vi "Main Tclk.vi"() -> ()   [LabVIEW 2018] (continued)
            n4773 = event-data() -> ("NewVal"=w4047:bool)  [unwired: 6 out]
            n4774 = case shown="True" w4047 {
              frame False {
              }
              frame True {
                n4775 = stacked-sequence {
                  frame #0 {
                    n4776 = local read "Last milling snapshot"() -> (w4051:path)
                    n4777 = local read "Last FIB recipe"() -> (w4057:path)
                    n4778 = local read "Re-engage Files"() -> (w4063:path)
                    n4779 = File/Directory Info(path=w4057) -> (path out=w4056:path, error out=w4052:errorcluster)  [unwired: 1 in, 5 out]
                    n4780 = Build Path(base path=w4063, name or relative path="pre.png") -> (appended path=w4061:path)
                    n4781 = File/Directory Info(path=w4051) -> (path out=w4050:path, error out=w4048:errorcluster)  [unwired: 1 in, 5 out]
                    n4782 = Unbundle By Name(w4052) -> ("status"=w4053:bool)
                    n4783 = Unbundle By Name(w4048) -> ("status"=w4049:bool)
                    n4784 = File/Directory Info(path=w4061) -> (error out=w4058:errorcluster)  [unwired: 1 in, 6 out]
                    n4785 = case shown="False" w4049 {
                      tunnel: w4050 -> [w4066 _]
                      tunnel: [w4065 w4069] -> w4060
                      tunnel: w4048 -> [_ w4069]
                      frame False {
                        n4786 = call-poly <vilib>:"Read From XML File.vi"("XML File Path"=w4066) -> ("error out"=w4064:errorcluster, "XML Elements"=w4067:string)  [unwired: 8 in, 1 out]
                        n4787 = Unflatten From XML(xml string=w4067, type=T47 {"Timestamp"=timestamp(0 s since 1904-01-01), "Double"=0.0, "FIB slice #"=0, "Reheat"=FALSE, "Double 2"=0.0, "Double 3"=0.0, "Double 4"=0.0} ("output cluster"), error in (no error)=w4064) -> (error out=w4065:errorcluster)  [unwired: 1 out]
                      }
                      frame True {
                      }
                    }
                    n4788 = case shown="False" w4053 {
                      tunnel: [w4071 w4073] -> w4059
                      tunnel: w4056 -> [w4070 _]
                      tunnel: w4052 -> [_ w4073]
                      frame False {
                        n4789 = call "Recipe read write.vi"("Write"=FALSE, "Recipe path"=w4070) -> ("error out"=w4071:errorcluster)  [unwired: 6 in, 3 out]
                      }
                      frame True {
                      }
                    }
                    n4790 = Merge Errors(w4060, w4059, w4058) -> (w4054:errorcluster)
                    n4791 = Unbundle By Name(w4054) -> ("status"=w4055:bool)
                    n4792 = local write "error out"(w4054) -> ()
                    n4793 = case shown="True" w4055 {
                      frame False {
                      }
                      frame True {
                        n4794 = local read "Milling para"() -> (w4076:T35)
                        n4795 = Two Button Dialog(message="Files needed for resume do not exist or are corrupted\nLoad information from the last good data file (*.dat)?") -> (T button?=w4074:bool)  [unwired: 2 in]
                        "dat to csv and xml" <- w4074
                        n4796 = Bundle By Name(cluster=w4076, "Mill start from Last"=w4074) -> (w4075:T35)
                        n4797 = local write "Milling para"(w4075) -> ()
                      }
                    }
                  }
                  frame #1 {
                    n4798 = local read "dat to csv and xml"() -> (w4078:bool)
                    n4799 = case shown="True" w4078 {
                      frame False {
                      }
                      frame True {
                        n4800 = call "File Dialog4"("start path"=path "E:/Images", "prompt"="Select the last good .dat file", "pattern (all files)"="*.dat" ("pattern label"), "pattern label"="Data file") -> ("selected path"=w4081:path, "cancelled"=w4079:bool, "error out"=w4084:errorcluster)  [unwired: 8 in, 1 out]
                        n4801 = local write "Read recipe path"(w4081) -> ()
                        n4802 = local write "error out"(w4084) -> ()
                        n4803 = case shown="True" w4079 {
                          frame False {
                            n4804 = local write "Load recipe"(TRUE ("Load recipe")) -> ()
                          }
                          frame True {
                            n4805 = local read "Milling para"() -> (w4087:T35)
                            n4806 = Bundle By Name(cluster=w4087, "Mill start from Last"=FALSE) -> (w4089:T35)
                            n4807 = local write "Milling para"(w4089) -> ()
                          }
                        }
                      }
                    }
                  }
                  frame #2 {
                    n4808 = local read "Milling para"() -> (w4091:T35)
                    n4809 = Unbundle By Name(w4091) -> ("Mill start from Last"=w4090:bool)
                    n4810 = case shown="True" w4090 {
                      frame False {
                      }
                      frame True {
                        n4811 = One Button Dialog(message="Resume from the last recipe and milling position ") -> ()  [unwired: 1 in, 1 out]
                      }
                    }
                  }
                }
              }
            }
          }
          event "Milling para.FIB PID reset": Value Change {
            n4812 = event-data() -> ("NewVal"=w4093:bool)  [unwired: 2 out]
            n4813 = shared-variable ".\\Zeiss Library.lvlib\\FIB PID reset"(w4093) -> ()  [unwired: 1 in, 1 out]
          }
          event "Milling para.FIB PID target": Value Change {
            n4814 = event-data() -> ()  [unwired: 7 out]
            n4815 = local read "Alert Settings"() -> (w4096:T36)
            n4816 = Bundle By Name(cluster=w4096, "FIB CL current alarm"=FALSE) -> (w4095:T36)
            n4817 = local write "Alert Settings"(w4095) -> ()
          }
          event "Pre image": Value Change {
            n4818 = event-data() -> ("NewVal"=w4097:bool)  [unwired: 2 out]
            n4819 = case shown="True" w4097 {
              frame False {
                n4820 = local write "Status message"("standby" ("Status message")) -> ()
                n4821 = shared-variable "My Computer\\Zeiss Library.lvlib\\Realtime Imaging stop"(TRUE ("Unfreeze")) -> ()  [unwired: 1 in, 1 out]
              }
              frame True {
                n4822 = stacked-sequence {
                  frame #0 {
                    n4823 = local read "FIB HW Config"() -> (w4108:T23)
                    n4824 = local read "FIB HW Config"() -> (w4105:T23)
                    n4825 = local write "Status message"("FIB Pre Imaging" ("Status message")) -> ()
                    n4826 = Unbundle By Name(w4108) -> ("Beam blank"=w4107:tag)
                    n4827 = Unbundle By Name(w4105) -> ("FIB Ext Scan"=w4103:tag)
                    n4828 = local read "Api"() -> (w4100:refnum<k7>)
                    n4829 = call "FIB beam blank.vi"("Api"=w4100, "Beam blanked"=TRUE, "lines"=w4107) -> ()  [unwired: 2 in, 1 out]
                    n4830 = call "FIB ext scan.vi"("Ext on"=TRUE ("data"), "FIB Ext Scan"=w4103) -> ()  [unwired: 9 in, 1 out]
                    n4831 = local write "Image Tabs"(T37."FIB Milling Offset after Pause" ("Image Tabs")) -> ()
                  }
                  frame #1 {
                    n4832 = local read "Machine Type"() -> (w4109:u8)
                    n4833 = case shown="1" w4109 {
                      frame 0, Default {
                      }
                      frame 1 {
                        w4112 = TRUE ("Close session")
                        n4834 = local read "COM port"() -> (w4114:refnum<visa-resource-name>)
                        n4835 = call "Remcon32 command.vi"("Initialization"=w4112, "SEM command"="edx 1", "COM port in"=w4114) -> ("COM port out"=w4113:refnum<visa-resource-name>)  [unwired: 5 in, 3 out]
                        n4836 = call "FIB mode.vi"("Close session"=w4112, "Iterations"=u32 3, "FIB mode"=T10."FIB", "COM port in"=w4113) -> ()  [unwired: 6 in, 2 out]
                      }
                    }
                  }
                  frame #2 {
                    n4837 = shared-variable ".\\Zeiss Library.lvlib\\Milling Z Voltage RT"() -> (w4117:sgl)  [unwired: 1 in, 1 out]
                    n4838 = local read "FIB Options"() -> (w4120:T33)
                    n4839 = local read "FIB Scan Parameters"() -> (w4124:T32)
                    n4840 = property on="Pre Image" class="IntGraph (strict)"() -> ("Width"=w4133:u32, "Height"=w4132:u32)  [unwired: 2 in, 2 out]
                    n4841 = local read "FIB Options"() -> (w4140:T33)
                    n4842 = local read "Milling para"() -> (w4123:T35)
                    n4843 = local read "FIB Scan Parameters"() -> (w4146:T32)
                    n4844 = expression code="x/1000"("FIB Y zoom pixel (nm)") -> (w4134:dbl)
                    n4845 = Decrement(x=w4132) -> (x-1=w4131:u32)
                    n4846 = Unbundle By Name(w4120) -> ("Flip z"=w4119:bool)
                    n4847 = Unbundle By Name(w4140) -> ("Flip x"=w4136:bool)
                    n4848 = Unbundle By Name(w4123) -> ("X offset (um)"=w4152:sgl, "X center (um)"=w4151:sgl, "FIB FOV (um)"=w4122:sgl)
                    n4849 = Multiply(x=w4134, y=w4131) -> (x*y=w4130:dbl)
                    "FIB Y zoom size (um)" <- w4130
                    n4850 = Unbundle By Name(w4124) -> ("Z size (V)"=w4125:dbl)
                    n4851 = Unbundle By Name(w4146) -> ("X size (V)"=w4141:dbl)
                    n4852 = Negate(x=w4117) -> (-x=w4118:sgl)
                    n4853 = Add(x=w4152, y=w4151) -> (x+y=w4153:sgl)
                    n4854 = Select(t=w4118, s=w4119, f=w4117) -> (s? t:f=w4116:sgl)
                    n4855 = Divide(x=w4116, y=w4125) -> (x/y=w4126:dbl)
                    n4856 = Multiply(x=w4126, y=w4122) -> (x*y=w4127:dbl)
                    n4857 = shared-variable ".\\Zeiss Library.lvlib\\Milling Z Voltage RT"() -> (w4149:sgl)  [unwired: 1 in, 1 out]
                    n4858 = call "Milling parameter to trapezoidal shape.vi"("Y location (um)"=w4127, "Milling para"=w4123) -> ("X size (um) @ Y"=w4121:dbl)  [unwired: 5 in, 4 out]
                    n4859 = expression code="x*1.2"(w4121) -> (w4128:dbl)
                    "FIB X zoom size (um)" <- w4128
                    n4860 = Divide(x=w4153, y=w4122) -> (x/y=w4142:sgl)
                    n4861 = Divide(x=w4128, y=w4122) -> (x/y=w4145:dbl)
                    n4862 = Multiply(x=w4142, y=w4141) -> (x*y=w4138:dbl)
                    n4863 = Multiply(x=w4145, y=w4141) -> (x*y=w4129:dbl)
                    n4864 = Multiply(x=w4141, y=w4130) -> (x*y=w4144:dbl)
                    n4865 = Negate(x=w4138) -> (-x=w4139:dbl)
                    n4866 = Divide(x=w4144, y=w4122) -> (x/y=w4143:dbl)
                    n4867 = Select(t=w4139, s=w4136, f=w4138) -> (s? t:f=w4137:dbl)
                    n4868 = local read "FIB Zoom Parameters"() -> (w4155:T34)
                    n4869 = Bundle By Name(cluster=w4155, "X resolution"=w4133, "Y resolution"=w4131, "X center"=w4137, "X size (V)"=w4129, "Y center"=w4149, "Y size (V)"=w4143, "Frame line rampdown ratio"=-0.1, "Scan rate (Hz)"=u32 200000, "Oversampling"=u16 20) -> (w4154:T34)
                    n4870 = local write "FIB Zoom Parameters"(w4154) -> ()
                  }
                  frame #3 {
                    n4871 = Wait (ms)(milliseconds to wait=u32 200) -> ()  [unwired: 1 out]
                  }
                  frame #4 {
                    w4158 = TRUE ("As subVi")
                    n4872 = local read "FIB HW Config"() -> (w4159:T23)
                    n4873 = local read "FIB Options"() -> (w4160:T33)
                    n4874 = call "FIB realtime imaging PXIe-6124.vi"("HW Config"=w4159, "Options"=w4160, "Single scan"=w4158, "Scan Para"="FIB Zoom Parameters", "As subVi"=w4158) -> ()  [unwired: 4 in, 2 out]
                  }
                  frame #5 {
                    n4875 = Wait (ms)(milliseconds to wait=u32 100) -> ()  [unwired: 1 out]
                    n4876 = local read "Milling para"() -> (w4166:T35)
                    n4877 = local read "FIB Zoom Parameters"() -> (w4161:T34)
                    n4878 = control-ref of="Pre Image"() -> (w4169:refnum<vi>)
                    n4879 = local read "FIB Scan Parameters"() -> (w4164:T32)
                    n4880 = local read "FIB Options"() -> (w4163:T33)
                    n4881 = shared-variable ".\\Zeiss Library.lvlib\\Milling Z Voltage RT"() -> (w4162:sgl)  [unwired: 1 in, 1 out]
                    n4882 = call "FIB zoom image draw milling.vi"("Milling Z voltage"=w4162, "Milling para"=w4166, "FIB Zoom Parameters"=w4161, "FIB Options"=w4163, "FIB Scan Parameters"=w4164, "Pre image"=TRUE, "Image reference"=w4169) -> ()  [unwired: 5 in]
                    n4883 = Unbundle By Name(w4166) -> ("X offset (um)"=→"X offset pre (um)":sgl, "Z offset (um)"=→"Y offset pre (um)":sgl)
                  }
                  frame #6 {
                    n4884 = local read "Pre Image"() -> (w4171:i16[][])
                    n4885 = Array Size(array=w4171) -> (size(s)=w4172:i32[])
                    n4886 = local write "Pre image"(FALSE ("Pre image")) -> ()
                    n4887 = local write "Status message"("standby" ("Status message")) -> ()
                    n4888 = Add Array Elements(numeric array=w4172) -> (sum=w4173:i32)
                    n4889 = Not Equal To 0?(x=w4173) -> (x != 0?=w4174:bool)
                    n4890 = case shown="True" w4174 {
                      tunnel: w4171 -> [_ w4179]
                      frame False {
                      }
                      frame True {
                        n4891 = local read "Last FIB zoom pre image"() -> (w4181:path)
                        n4892 = call "16bit Image Normalization.vi"("Transpose"=FALSE, "Input image"=w4179) -> ("Normalized image"=w4178:u8[][])  [unwired: 5 in, 4 out]
                        n4893 = call <vilib>:"Flatten Pixmap.vi"("colors"=u32[] [16777222, 65793, 131586, 197379, 263172, 328965, 394758, 460551, 526344, 592137, 657930, 723723, 789516, 855309, 921102, 986895, 1052688, 1118481, 1184274, 1250067, 1315860, 1381653, 1447446, 1513239, 1579032, 1644825, 1710618, 1776411, 1842204, 1907997, 1973790, 2039583, 2105376, 2171169, 2236962, 2302755, 2368548, 2434341, 2500134, 2565927, 2631720, 2697513, 2763306, 2829099, 2894892, 2960685, 3026478, 3092271, 3158064, 3223857, 3289650, 3355443, 3421236, 3487029, 3552822, 3618615, 3684408, 3750201, 3815994, 3881787, 3947580, 4013373, 4079166, 4144959, 4210752, 4276545, 4342338, 4408131, 4473924, 4539717, 4605510, 4671303, 4737096, 4802889, 4868682, 4934475, 5000268, 5066061, 5131854, 5197647, 5263440, 5329233, 5395026, 5460819, 5526612, 5592405, 5658198, 5723991, 5789784, 5855577, 5921370, 5987163, 6052956, 6118749, 6184542, 6250335, 6316128, 6381921, 6447714, 6513507, 6579300, 6645093, 6710886, 6776679, 6842472, 6908265, 6974058, 7039851, 7105644, 7171437, 7237230, 7303023, 7368816, 7434609, 7500402, 7566195, 7631988, 7697781, 7763574, 7829367, 7895160, 7960953, 8026746, 8092539, 8158332, 8224125, 8289918, 8355711, 8421504, 8487297, 8553090, 8618883, 8684676, 8750469, 8816262, 8882055, 8947848, 9013641, 9079434, 9145227, 9211020, 9276813, 9342606, 9408399, 9474192, 9539985, 9605778, 9671571, 9737364, 9803157, 9868950, 9934743, 10000536, 10066329, 10132122, 10197915, 10263708, 10329501, 10395294, 10461087, 10526880, 10592673, 10658466, 10724259, 10790052, 10855845, 10921638, 10987431, 11053224, 11119017, 11184810, 11250603, 11316396, 11382189, 11447982, 11513775, 11579568, 11645361, 11711154, 11776947, 11842740, 11908533, 11974326, 12040119, 12105912, 12171705, 12237498, 12303291, 12369084, 12434877, 12500670, 12566463, 12632256, 12698049, 12763842, 12829635, 12895428, 12961221, 13027014, 13092807, 13158600, 13224393, 13290186, 13355979, 13421772, 13487565, 13553358, 13619151, 13684944, 13750737, 13816530, 13882323, 13948116, 14013909, 14079702, 14145495, 14211288, 14277081, 14342874, 14408667, 14474460, 14540253, 14606046, 14671839, 14737632, 14803425, 14869218, 14935011, 15000804, 15066597, 15132390, 15198183, 15263976, 15329769, 15395562, 15461355, 15527148, 15592941, 15658734, 15724527, 15790320, 15856113, 15921906, 15987699, 16053492, 16119285, 16185078, 16250871, 16316664, 16382457, 16448250, 16514043, 16579836, 16645629, 16711422, 16448250] ("256 gray scale"), "8-bit pixmap"=w4178) -> ("image data"=w4180:T55)  [unwired: 4 in, 5 out]
                        n4894 = call <vilib>:"Write PNG File.vi"("image data"=w4180, "path to PNG file"=w4181) -> ()  [unwired: 1 in, 9 out]
                      }
                    }
                  }
                }
              }
            }
          }
          event "Post image": Value Change {
            n4895 = event-data() -> ("NewVal"=w4183:bool)  [unwired: 2 out]
            n4896 = case shown="True" w4183 {
              frame False {
                n4897 = local write "Status message"("standby" ("Status message")) -> ()
                n4898 = shared-variable "My Computer\\Zeiss Library.lvlib\\Realtime Imaging stop"(TRUE ("Unfreeze")) -> ()  [unwired: 1 in, 1 out]
              }
              frame True {
                n4899 = stacked-sequence {
                  frame #0 {
                    n4900 = local read "FIB HW Config"() -> (w4194:T23)
                    n4901 = local read "FIB HW Config"() -> (w4191:T23)
                    n4902 = local write "Status message"("FIB Post Imaging" ("Status message")) -> ()
                    n4903 = Unbundle By Name(w4194) -> ("Beam blank"=w4193:tag)
                    n4904 = Unbundle By Name(w4191) -> ("FIB Ext Scan"=w4189:tag)
                    n4905 = local read "Api"() -> (w4186:refnum<k7>)
                    n4906 = call "FIB beam blank.vi"("Api"=w4186, "Beam blanked"=TRUE, "lines"=w4193) -> ()  [unwired: 2 in, 1 out]
                    n4907 = call "FIB ext scan.vi"("Ext on"=TRUE ("data"), "FIB Ext Scan"=w4189) -> ()  [unwired: 9 in, 1 out]
                    n4908 = local write "Image Tabs"(T37."FIB Milling Offset after Pause" ("Image Tabs")) -> ()
                  }
                  frame #1 {
                    n4909 = local read "Machine Type"() -> (w4195:u8)
                    n4910 = case shown="1" w4195 {
                      frame 0, Default {
                      }
                      frame 1 {
                        w4198 = TRUE ("Close session")
                        n4911 = local read "COM port"() -> (w4200:refnum<visa-resource-name>)
                        n4912 = call "Remcon32 command.vi"("Initialization"=w4198, "SEM command"="edx 1", "COM port in"=w4200) -> ("COM port out"=w4199:refnum<visa-resource-name>)  [unwired: 5 in, 3 out]
                        n4913 = call "FIB mode.vi"("Close session"=w4198, "Iterations"=u32 3, "FIB mode"=T10."FIB", "COM port in"=w4199) -> ()  [unwired: 6 in, 2 out]
                      }
                    }
                  }
                  frame #2 {
                    n4914 = local read "FIB Y zoom pixel (nm)"() -> (w4222:dbl)
                    n4915 = property on="Pre Image" class="IntGraph (strict)"() -> ("Height"=w4221:u32)  [unwired: 2 in, 2 out]
                    n4916 = local read "FIB Scan Parameters"() -> (w4218:T32)
                    n4917 = local read "Milling para"() -> (w4219:T35)
                    n4918 = local read "FIB Zoom Parameters"() -> (w4204:T34)
                    n4919 = shared-variable ".\\Zeiss Library.lvlib\\Milling Z Voltage RT"() -> (w4203:sgl)  [unwired: 1 in, 1 out]
                    n4920 = Decrement(x=w4221) -> (x-1=w4212:u32)
                    n4921 = Unbundle By Name(w4219) -> ("FIB FOV (um)"=w4220:sgl)
                    n4922 = Unbundle By Name(w4218) -> ("X size (V)"=w4217:dbl)
                    n4923 = expression code="x/1000"(w4222) -> (w4213:dbl)
                    n4924 = Unbundle By Name(w4204) -> ("Y size (V)"=w4209:dbl)
                    n4925 = Bundle By Name(cluster=w4204, "Y center"=w4203) -> (w4202:T34)
                    n4926 = Multiply(x=w4212, y=w4217) -> (x*y=w4216:dbl)
                    n4927 = Divide(x=w4216, y=w4220) -> (x/y=w4215:dbl)
                    n4928 = local write "FIB Zoom Parameters"(w4202) -> ()
                    n4929 = Divide(x=w4209, y=w4215) -> (x/y=w4214:dbl)
                    n4930 = Multiply(x=w4213, y=w4215) -> (x*y=w4210:dbl)
                    n4931 = Subtract(x=w4210, y=w4209) -> (x-y=w4206:dbl)
                    n4932 = Multiply(x=w4213, y=w4212) -> (x*y=w4211:dbl)
                    n4933 = Absolute Value(x=w4206) -> (abs(x)=w4205:dbl)
                    n4934 = Greater?(x=w4205, y=0.0001) -> (0:w4208:bool)
                    n4935 = case shown="True" w4208 {
                      tunnel: w4210 -> [_ w4228]
                      tunnel: w4214 -> [_ w4225]
                      tunnel: w4211 -> [_ w4223]
                      frame False {
                      }
                      frame True {
                        n4936 = expression code="x*1000"(w4225) -> (w4224:dbl)
                        n4937 = Two Button Dialog(message="Y pixel was modified since the last pre image was taken", 1:"Continue with new value" ("T button name (\"OK\")"), 2:"Use old value" ("T button name (\"OK\")")) -> (T button?=w4229:bool)
                        n4938 = case shown="True" w4229 {
                          tunnel: w4228 -> [w4232 _]
                          tunnel: w4224 -> [_ w4235]
                          tunnel: w4223 -> [w4231 _]
                          frame False {
                            n4939 = local read "FIB Zoom Parameters"() -> (w4234:T34)
                            n4940 = Bundle By Name(cluster=w4234, "Y size (V)"=w4232) -> (w4233:T34)
                            n4941 = local write "FIB Zoom Parameters"(w4233) -> ()
                            n4942 = local write "FIB Y zoom size (um)"(w4231) -> ()
                          }
                          frame True {
                            n4943 = local write "FIB Y zoom pixel (nm)"(w4235) -> ()
                          }
                        }
                      }
                    }
                  }
                  frame #3 {
                    w4237 = TRUE ("As subVi")
                    n4944 = local read "FIB Zoom Parameters"() -> (w4236:T34)
                    n4945 = local read "FIB HW Config"() -> (w4238:T23)
                    n4946 = local read "FIB Options"() -> (w4239:T33)
                    n4947 = call "FIB realtime imaging PXIe-6124.vi"("HW Config"=w4238, "Options"=w4239, "Single scan"=w4237, "Scan Para"=w4236, "As subVi"=w4237) -> ()  [unwired: 4 in, 2 out]
                  }
                  frame #4 {
                    n4948 = Wait (ms)(milliseconds to wait=u32 100) -> ()  [unwired: 1 out]
                  }
                  frame #5 {
                    n4949 = local read "FIB Zoom Parameters"() -> (w4266:T34)
                    n4950 = local read "X offset pre (um)"() -> (w4242:dbl)
                    n4951 = local read "Y offset pre (um)"() -> (w4241:dbl)
                    n4952 = local read "Post Image"() -> (w4255:i16[][])
                    n4953 = local read "Pre Image"() -> (w4254:i16[][])
                    n4954 = call "Image Alignment.vi"("Image 2"=w4254, "Image 1"=w4255) -> ("Y shift"=w4258:i32, "X shift"=w4263:i32)  [unwired: 7 in, 1 out]
                    n4955 = Unbundle By Name(w4266) -> ("X resolution"=w4262:u32, "Y resolution"=w4257:u32, "X size (V)"=w4261:dbl, "Y size (V)"=w4256:dbl)
                    n4956 = Divide(x=w4263, y=w4262) -> (x/y=w4259:dbl)
                    n4957 = Divide(x=w4258, y=w4257) -> (x/y=w4260:dbl)
                    n4958 = local read "Milling para"() -> (w4265:T35)
                    n4959 = local read "FIB Scan Parameters"() -> (w4264:T32)
                    n4960 = Multiply(x=w4259, y=w4261) -> (x*y=w4250:dbl)
                    n4961 = Multiply(x=w4260, y=w4256) -> (x*y=w4251:dbl)
                    n4962 = Unbundle By Name(w4265) -> ("FIB FOV (um)"=w4253:sgl)
                    n4963 = Unbundle By Name(w4264) -> ("X size (V)"=w4252:dbl)
                    n4964 = Divide(x=w4253, y=w4252) -> (x/y=w4249:dbl)
                    n4965 = Multiply(x=w4250, y=w4249) -> (x*y=w4246:dbl)
                    n4966 = Multiply(x=w4251, y=w4249) -> (x*y=w4244:dbl)
                    n4967 = Add(x=w4246, y=w4242) -> (x+y=w4245:dbl)
                    n4968 = Add(x=w4244, y=w4241) -> (x+y=w4243:dbl)
                    n4969 = local read "Milling para"() -> (w4248:T35)
                    n4970 = Bundle By Name(cluster=w4248, "X offset (um)"=w4245, "Z offset (um)"=w4243) -> (w4247:T35)
                    n4971 = local write "Milling para"(w4247) -> ()
                  }
                  frame #6 {
                    n4972 = local read "X offset pre (um)"() -> (w4269:dbl)
                    n4973 = local read "Y offset pre (um)"() -> (w4268:dbl)
                    n4974 = local read "Milling para"() -> (w4274:T35)
                    n4975 = local read "FIB Zoom Parameters"() -> (w4267:T34)
                    n4976 = control-ref of="Post Image"() -> (w4275:refnum<vi>)
                    n4977 = local read "FIB Scan Parameters"() -> (w4272:T32)
                    n4978 = local read "FIB Options"() -> (w4271:T33)
                    n4979 = shared-variable ".\\Zeiss Library.lvlib\\Milling Z Voltage RT"() -> (w4270:sgl)  [unwired: 1 in, 1 out]
                    n4980 = call "FIB zoom image draw milling.vi"("Milling Z voltage"=w4270, "Milling para"=w4274, "Z offset pre (um)"=w4268, "X offset pre (um)"=w4269, "FIB Zoom Parameters"=w4267, "FIB Options"=w4271, "FIB Scan Parameters"=w4272, "Pre image"=FALSE, "Image reference"=w4275) -> ()  [unwired: 3 in]
                  }
                  frame #7 {
                    n4981 = local write "Post image"(FALSE ("Pre image")) -> ()
                    n4982 = local write "Status message"("standby" ("Status message")) -> ()
                  }
                }
              }
            }
          }
          event "Hardware Configuration.Save config file": Value Change {
            # "THIS VI WRITES ALL THE HARDWARE CONFIG TAB CONTROLS TO THE .INI FILE."
            n4983 = event-data() -> ()  [unwired: 2 out]
            n4984 = disable-structure shown="Disabled" {
              frame Disabled {
                n4985 = stacked-sequence {
                  frame #0 {
                    n4986 = local read "HW config items"() -> (w4281:string[])
                    n4987 = local read "Hardware Configuration"() -> (w4285:T25)
                    n4988 = local read "Detector Information"() -> (w4286:T8)
                    n4989 = local read "Hardware Configuration"() -> (w4283:T25)
                    n4990 = Unbundle By Name(w4285) -> ("Machine ID"=w4294:string, "Machine Type"=w4300:u8, "SEM Max FOV (um)"=w4287:sgl, "Det min (V)"=w4288:dbl, "Det max (V)"=w4289:dbl)
                    n4991 = Unbundle By Name(w4286) -> ("Brightness A"=w4291:dbl, "Contrast A"=w4290:dbl, "Detector B name"=w4295:string, "Brightness B"=w4292:dbl, "Contrast B"=w4293:dbl)
                    n4992 = Unbundle By Name(w4283) -> ("Configuration file"=w4282:path)
                    n4993 = Build Array(w4287, w4288, w4289, w4291, w4290) -> (w4296:dbl[])
                    n4994 = Build Array(w4292, w4293) -> (w4298:dbl[])
                    n4995 = case shown="2" w4300 {
                      tunnel: ["Feiss" ("Machine ID") "NVision" ("Machine ID") "Jeiss" ("Machine ID")] -> w4301
                      frame 0, Default {
                      }
                      frame 1 {
                      }
                      frame 2 {
                      }
                    }
                    n4996 = for {
                      tunnel: w4296 -> [w4322] mode=indexing
                      tunnel: [w4321] -> w4297 mode=indexing
                      n4997 = Format Into String(w4322) -> (resulting string=w4321:string)  [unwired: 3 in, 1 out]
                    }
                    n4998 = for {
                      tunnel: w4298 -> [w4320] mode=indexing
                      tunnel: [w4319] -> w4299 mode=indexing
                      n4999 = Format Into String(w4320) -> (resulting string=w4319:string)  [unwired: 3 in, 1 out]
                    }
                    n5000 = Build Array (concatenate)(w4294, w4301, w4297, w4295, w4299) -> (w4302:string[])
                    n5001 = for {
                      tunnel: w4281 -> [w4315] mode=indexing
                      tunnel: w4302 -> [w4313] mode=indexing
                      tunnel: [w4312] -> w4284 mode=indexing
                      n5002 = Concatenate Strings(w4315, "," ("string"), w4313) -> (w4312:string)
                    }
                    n5003 = Build Path(name or relative path=w4282) -> (appended path=w4305:path)  [unwired: 1 in]
                    n5004 = Open/Create/Replace File(file path (use dialog)=w4305, operation (0:open)=T49."replace or create with confirmation") -> (refnum out=w4307:refnum<file>, error out=w4308:errorcluster)  [unwired: 1 in, 4 out]
                    n5005 = Set File Position(refnum=w4307, from (0:start)=enum16{"start", "end", "current"}."end", error in=w4308) -> (refnum out=w4309:refnum<file>, error out=w4306:errorcluster)  [unwired: 1 out]
                    n5006 = Write to Text File(file (use dialog)=w4309, text=w4284, error in=w4306) -> (refnum out=w4310:refnum<file>, error out=w4311:errorcluster)  [unwired: 2 out]
                    n5007 = Close File(refnum=w4310, error in=w4311) -> ()  [unwired: 2 out]
                  }
                  frame #1 {
                    n5008 = local read "Hardware Configuration"() -> (w4325:T25)
                    n5009 = Bundle By Name(cluster=w4325, "Save config file"=FALSE) -> (w4324:T25)
                    n5010 = local write "Hardware Configuration"(w4324) -> ()
                  }
                }
              }
              frame Enabled {
              }
            }
            n5011 = local read "Hardware Configuration"() -> (w4280:T25)
            n5012 = Bundle By Name(cluster=w4280, "Save config file"=FALSE) -> (w4279:T25)
            n5013 = local write "Hardware Configuration"(w4279) -> ()
            n5014 = call "Write Config Settings to INI file.vi"("Hardware Configuration"=w4279) -> ()  [unwired: 11 in]
          }
          event "File Information.Save recipe": Value Change {
            n5015 = event-data() -> ()  [unwired: 2 out]
            n5016 = stacked-sequence {
              frame #0 {
              }
              frame #1 {
                n5017 = call "File Dialog"("start path"=path "E:/Recipes", "prompt"="Select an existing recipe to \noverwrite or a directory for \nthe new recipe") -> ("selected path"=w4328:path, "cancelled"=w4330:bool, "error out"=→"error out":errorcluster)  [unwired: 10 in, 1 out]
                n5018 = case shown="False" w4330 {
                  tunnel: w4328 -> [w4337 _]
                  frame False {
                    n5019 = Strip Path(path=w4337) -> (name=w4333:string)  [unwired: 1 out]
                    n5020 = xnode "Match Regular Expression"("input string"=w4333, "regular expression"=".csv") -> ("offset past match"=w4335:i32)  [unwired: 4 in, 4 out]
                    n5021 = Equal?(x=w4335, y=-1) -> (x = y?=w4334:bool)
                    n5022 = case shown="True" w4334 {
                      tunnel: [w4340 w4341] -> w4339
                      tunnel: w4333 -> [w4340 _]
                      frame False {
                      }
                      frame True {
                        n5023 = call "Recipe File Name"() -> ("FIB-SEM recipe YY-MM-DD <user input>.csv"=w4341:string)  [unwired: 17 in, 2 out]
                      }
                    }
                    n5024 = local read "Recipe input"() -> (w4331:T7)
                    n5025 = call "Recipe read write.vi"("Write"=TRUE, "Info"=w4339, "Recipe path"=w4337, "Write input"=w4331) -> ()  [unwired: 4 in, 4 out]
                  }
                  frame True {
                  }
                }
              }
              frame #2 {
                n5026 = Wait (ms)(milliseconds to wait=u32 200) -> ()  [unwired: 1 out]
              }
              frame #3 {
                n5027 = local read "File Information"() -> (w4456:T31)
                n5028 = Bundle By Name(cluster=w4456, "Save recipe"=FALSE ("Save config file")) -> (w4455:T31)
                n5029 = local write "File Information"(w4455) -> ()
              }
            }
          }
          event "File Information.Load recipe": Value Change {
            n5030 = event-data() -> ()  [unwired: 2 out]
            n5031 = stacked-sequence {
              tunnel: [w4460 _ _] -> w4458
              tunnel: w4457 -> [w4459 _ _]
              frame #0 {
                n5032 = call "File Dialog2"("start path"=path "E:/images", "prompt"="Select the recipe", "pattern (all files)"="*.csv;*.dat" ("pattern label"), "pattern label"="Recipe or Data file") -> ("selected path"=w4464:path, "cancelled"=w4465:bool, "error out"=w4466:errorcluster)  [unwired: 8 in, 1 out]
                n5033 = local write "error out"(w4466) -> ()
                n5034 = case shown="False" w4465 {
                  tunnel: w4464 -> [w4469 _]
                  tunnel: [w4468 w4497] -> w4460
                  tunnel: w4459 -> [_ w4497]
                  frame False {
                    n5035 = stacked-sequence {
                      tunnel: w4469 -> [w4471 _ _]
                      tunnel: [_ _ w4496] -> w4468
                      frame #0 {
                        n5036 = local write "Read recipe path"(w4471) -> ()
                        n5037 = Strip Path(path=w4471) -> (name=w4474:string)  [unwired: 1 out]
                        n5038 = Match Pattern(string=w4474, regular expression=".dat") -> (offset past match=w4473:i32)  [unwired: 1 in, 3 out]
                        n5039 = Not Equal?(x=w4473, y=-1) -> (x != y?=w4470:bool)
                        n5040 = case shown="True" w4470 {
                          tunnel: w4471 -> [_ w4493]
                          frame False {
                          }
                          frame True {
                            n5041 = call "Zeiss File Header Tclk.vi"("Write"=FALSE, "Input file path"=w4493) -> ("Ouputs"=w4492:T79)  [unwired: 7 in, 2 out]
                            n5042 = Unbundle By Name(w4492) -> ("SEM parameters"=w4491:T13, "FIB parameters"=w4490:T80, "Data Logging"=w4488:T81)
                            n5043 = Unbundle By Name(w4488) -> ("Temp (F)"=w4487:sgl, "FIB Faraday Cup (nA)"=w4486:sgl, "FIB Specimen I (nA)"=w4485:sgl, "Beam Dump 1 (nA)"=w4484:sgl, "Beam Dump 2 (nA)"=w4477:sgl, "Milling I (nA)"=w4476:sgl, "SEM Specimen I (nA)"=w4479:sgl, "Milling Z voltage (V)"=w4483:sgl, "Focus Index"=w4482:sgl, "FIB slice #"=w4481:u32)
                            n5044 = local write "SEM Parameters"(w4491) -> ()
                            n5045 = local write "FIB Parameters"(w4490) -> ()
                            n5046 = local write "Temp (F)"(w4487) -> ()
                            n5047 = local write "Faraday Cup (nA)"(w4486) -> ()
                            n5048 = local write "Specimen I (nA)"(w4485) -> ()
                            n5049 = local write "Beam Dump 1 (nA)"(w4484) -> ()
                            n5050 = local write "Beam Dump 2 (nA)"(w4477) -> ()
                            n5051 = local write "Milling I (nA)"(w4476) -> ()
                            n5052 = local write "Milling Z voltage (V)"(w4483) -> ()
                            n5053 = local write "Focus Index"(w4482) -> ()
                            n5054 = local write "FIB slice #"(w4481) -> ()
                            n5055 = local read "SEM Status"() -> (w4480:T12)
                            n5056 = Bundle By Name(cluster=w4480, "SEM Spec. I (nA)"=w4479) -> (w4478:T12)
                            n5057 = local write "SEM Status"(w4478) -> ()
                          }
                        }
                      }
                      frame #1 {
                        n5058 = local write "Load recipe"(TRUE ("Load recipe")) -> ()
                        n5059 = Wait (ms)(milliseconds to wait=u32 500) -> ()  [unwired: 1 out]
                      }
                      frame #2 {
                        n5060 = local read "Trapezoidal"() -> (w4496:cluster{"X":i16, "Y":i16}[])
                      }
                    }
                  }
                  frame True {
                  }
                }
              }
              frame #1 {
                n5061 = Wait (ms)(milliseconds to wait=u32 200) -> ()  [unwired: 1 out]
              }
              frame #2 {
                n5062 = local read "File Information"() -> (w4501:T31)
                n5063 = Bundle By Name(cluster=w4501, "Load recipe"=FALSE ("Save config file")) -> (w4500:T31)
                n5064 = local write "File Information"(w4500) -> ()
              }
            }
          }
          event "Clear": Value Change {
            n5065 = event-data() -> ()  [unwired: 7 out]
            n5066 = local read "Sample rate (Hz)"() -> (w4502:dbl)
            n5067 = Get Date/Time In Seconds() -> (seconds since 1Jan1904=w4505:timestamp)
            n5068 = Reciprocal(x=w4502) -> (1/x=w4503:dbl)
            n5069 = To Double Precision Float(number=w4505) -> (double precision float=w4504:dbl)
            n5070 = property on="Measurements" class="WFChart (strict)"("History Data"=dbl[][] [], "XScale.Offset"=w4504, "XScale.Multiplier"=w4503) -> ()  [unwired: 2 in, 2 out]
          }
          event "Alert Settings.Temperature alarm": Value Change {
            n5071 = event-data() -> ("NewVal"=w4507:bool)  [unwired: 6 out]
            n5072 = local write "Temperature warning armed"(w4507) -> ()
          }
          event "Alert Settings.SW error warning": Value Change {
            n5073 = event-data() -> ("NewVal"=w4508:bool)  [unwired: 6 out]
            n5074 = local write "SW error warning armed"(w4508) -> ()
          }
          event "Alert Settings.Focus index warning": Value Change {
            n5075 = event-data() -> ("NewVal"=w4509:bool)  [unwired: 6 out]
            n5076 = local write "Focus index warning armed"(w4509) -> ()
          }
          event "Alert Settings": Value Change {
            n5077 = event-data() -> ()  [unwired: 7 out]
            n5078 = local write "Continued fine milling frames"(-5 ("Continued fine milling frames")) -> ()
          }
          event "Coarse milling": Value Change {
            n5079 = event-data() -> ("NewVal"=w4511:bool)  [unwired: 6 out]
            n5080 = case shown="True" w4511 {
              frame False {
              }
              frame True {
                n5081 = Two Button Dialog(message="Quick settings for coarse milling:\n1. Disable certain alarms\n2. Enable low mag scan for every single high mag\n3. Reset image center and shifts to 0\n4. Reset to single tile\n5. Turn off file upload") -> (T button?=w4512:bool)  [unwired: 2 in]
                n5082 = case shown="True" w4512 {
                  frame False {
                    n5083 = local write "Coarse milling"(FALSE ("Coarse milling")) -> ()
                  }
                  frame True {
                    w4528 = sgl[] [0.0] ("dX (um)")
                    w4529 = u8 1 ("X tiles")
                    w4530 = TRUE ("Low mag scan")
                    w4534 = sgl 0.0 ("X center (um)")
                    w4536 = FALSE ("Upload")
                    n5084 = local read "SEM Scan Parameters"() -> (w4520:T26)
                    n5085 = local read "Low Mag SEM"() -> (w4533:T30)
                    n5086 = Bundle By Name(cluster=w4533, "Low mag scan"=w4530, "Low mag interval"=u32 1, "Show HM box"=w4530) -> (w4532:T30)
                    n5087 = Unbundle By Name(w4520) -> ("X stig"=w4527:sgl[][], "Y stig"=w4526:sgl[][], "X aln"=w4525:sgl[][], "Y aln"=w4524:sgl[][], "WD (mm)"=w4523:sgl[][])
                    n5088 = local write "Low Mag SEM"(w4532) -> ()
                    n5089 = Build Array(w4527, w4526, w4525, w4524, w4523) -> (w4522:sgl[][][])
                    n5090 = for {
                      tunnel: [w4545] -> w4521 mode=indexing
                      workers-P: _ -> [_]
                      tunnel: w4522 -> [w4541] mode=indexing
                      w4544 = 1 ("dimension size")
                      n5091 = Array Size(array=w4541) -> (size(s)=w4543:i32[])
                      n5092 = Multiply Array Elements(1:w4543) -> (0:w4542:i32)
                      n5093 = Reshape Array(w4541, w4542) -> (w4547:sgl[])
                      n5094 = call-poly <vilib>:"Mean.vi"("X"=w4547) -> ("mean"=w4546:dbl)  [unwired: 1 out]
                      n5095 = Initialize Array(w4546, w4544, w4544) -> (w4545:dbl[][])
                    }
                    n5096 = local read "Alert Settings"() -> (w4540:T36)
                    n5097 = Bundle By Name(cluster=w4540, "Specimen @ SEM alarm"=w4536, "FIB CL current alarm"=w4536, "Milling Z voltage alarm"=w4536, "Detector over scale warning"=w4536, "Focus index warning"=w4536) -> (w4539:T36)
                    n5098 = local read "SEM Options"() -> (w4538:T27)
                    n5099 = Bundle By Name(cluster=w4538, "Upload"=w4536) -> (w4537:T27)
                    n5100 = Index Array(array=w4521) -> (element #1=w4519:dbl[][], element #2=w4518:dbl[][], element #3=w4517:dbl[][], element #4=w4516:dbl[][], element #5=w4515:dbl[][])  [unwired: 15 in]
                    n5101 = local write "Alert Settings"(w4539) -> ()
                    n5102 = local write "SEM Options"(w4537) -> ()
                    n5103 = Bundle By Name(cluster=w4520, "X stig"=w4519, "Y stig"=w4518, "X aln"=w4517, "Y aln"=w4516, "WD (mm)"=w4515, "X tiles"=w4529, "Y tiles"=w4529, "dX (um)"=w4528, "dY (um)"=w4528, "X center (um)"=w4534, "Y center (um)"=w4534) -> (w4535:T26)
                    n5104 = local write "X shift (nm/image)"(w4534) -> ()
                    n5105 = local write "Y shift (nm/image)"(w4534) -> ()
                    n5106 = local write "SEM Scan Parameters"(w4535) -> ()
                  }
                }
              }
            }
          }
          event "SEM Options.Save": Value Change {
            n5107 = event-data() -> ("NewVal"=w4548:bool)  [unwired: 6 out]
            n5108 = case shown="False" w4548 {
              frame False {
                n5109 = local read "SEM Options"() -> (w4551:T27)
                n5110 = Bundle By Name(cluster=w4551, "Upload"=FALSE) -> (w4549:T27)
                n5111 = local write "SEM Options"(w4549) -> ()
              }
              frame True {
              }
            }
          }
          event "SEM Options.Upload": Value Change {
            n5112 = event-data() -> ("OldVal"=w4552:bool, "NewVal"=w4555:bool)  [unwired: 5 out]
            n5113 = local read "FIB"() -> (w4553:bool)
            n5114 = case shown="True" w4553 {
              tunnel: [TRUE ("T button?") w4557] -> w4554
              frame False {
              }
              frame True {
                n5115 = Two Button Dialog(message="Are you sure to change the  file upload settings?") -> (T button?=w4557:bool)  [unwired: 2 in]
              }
            }
            n5116 = case shown="True" w4554 {
              tunnel: w4555 -> [_ w4563]
              tunnel: w4552 -> [w4559 _]
              frame False {
                n5117 = local read "SEM Options"() -> (w4561:T27)
                n5118 = Bundle By Name(cluster=w4561, "Upload"=w4559) -> (w4560:T27)
                n5119 = local write "SEM Options"(w4560) -> ()
              }
              frame True {
                n5120 = case shown="True" w4563 {
                  frame False {
                  }
                  frame True {
                    n5121 = local read "SEM Options"() -> (w4570:T27)
                    n5122 = Bundle By Name(cluster=w4570, "Save"=TRUE ("Upload")) -> (w4568:T27)
                    n5123 = local write "SEM Options"(w4568) -> ()
                  }
                }
                n5124 = local read "Initial Options"() -> (w4564:T27)
                n5125 = Bundle By Name(cluster=w4564, "Upload"=w4563) -> (w4562:T27)
                n5126 = Select(t=T44."Enabled" ("Disabled"), s=w4563, f=T44."Disabled and Grayed Out" ("Disabled")) -> (s? t:f=w4567:T44)
                n5127 = local write "Initial Options"(w4562) -> ()
                n5128 = property on="Delete after upload" class="Bool (strict)"("DisabledEnum"=w4567) -> ()  [unwired: 2 in, 2 out]
              }
            }
          }
          event "SEM Options.8-bit": Value Change {
            n5129 = event-data() -> ("OldVal"=w4571:bool, "NewVal"=w4574:bool)  [unwired: 5 out]
            n5130 = local read "FIB"() -> (w4572:bool)
            n5131 = case shown="True" w4572 {
              tunnel: [TRUE ("T button?") w4576] -> w4573
              frame False {
              }
              frame True {
                n5132 = Two Button Dialog(message="Are you sure to change the  data type settings?") -> (T button?=w4576:bool)  [unwired: 2 in]
              }
            }
            n5133 = case shown="True" w4573 {
              tunnel: w4574 -> [_ w4582]
              tunnel: w4571 -> [w4578 _]
              frame False {
                n5134 = local read "SEM Options"() -> (w4580:T27)
                n5135 = Bundle By Name(cluster=w4580, "8-bit"=w4578) -> (w4579:T27)
                n5136 = local write "SEM Options"(w4579) -> ()
              }
              frame True {
                n5137 = local read "Initial Options"() -> (w4583:T27)
                n5138 = Bundle By Name(cluster=w4583, "8-bit"=w4582) -> (w4581:T27)
                n5139 = local write "Initial Options"(w4581) -> ()
              }
            }
          }
          event "Manual Upload": Value Change {
            n5140 = event-data() -> ()  [unwired: 7 out]
            n5141 = stacked-sequence {
              frame #0 {
                n5142 = local write "Manual Upload"(FALSE ("Manual Upload")) -> ()
              }
              frame #1 {
                n5143 = call "Enter sample ID and select options"() -> ("Delete after upload"=w4585:bool, "Sample ID"=w4586:string, "Next"=w4587:bool)  [unwired: 16 in, 1 out]
                n5144 = case shown="True" w4587 {
                  tunnel: w4586 -> [_ w4591]
                  tunnel: w4585 -> [_ w4590]
                  frame False {
                  }
                  frame True {
                    n5145 = local read "File Information"() -> (w4593:T31)
                    n5146 = Unbundle By Name(w4593) -> ("File path"=w4594:path)
                    n5147 = call "File Dialog3"("start path"=w4594, "prompt"="Select SEM Files to Upload", "pattern (all files)"="*.dat" ("pattern label")) -> ("selected paths"=w4592:path[], "cancelled"=w4589:bool, "error out"=w4588:errorcluster)  [unwired: 9 in, 1 out]
                    n5148 = local write "error out"(w4588) -> ()
                    n5149 = case shown="False" w4589 {
                      tunnel: w4592 -> [w4599 _]
                      tunnel: w4591 -> [w4598 _]
                      tunnel: w4590 -> [w4597 _]
                      frame False {
                        n5150 = for {
                          tunnel: w4599 -> [w4603] mode=indexing
                          tunnel: w4598 -> [w4602]
                          tunnel: w4597 -> [w4601]
                          w4611 = "^" ("replace string (\"\")")
                          w4619 = T82 3 items=["no dialog", "OK message", "continue or stop message", "OK message + warnings", "continue/stop + warnings"] ("type of dialog (OK msg:1)")
                          n5151 = shared-variable ".\\Zeiss Library.lvlib\\Upload flags path"() -> (w4600:string)  [unwired: 1 in, 1 out]
                          n5152 = String To Path(string=w4600) -> (path=w4626:path)
                          n5153 = Path To String(path=w4603) -> (string=w4614:string)
                          n5154 = File/Directory Info(path=w4626) -> (path out=w4623:path, error out=w4625:errorcluster)  [unwired: 1 in, 5 out]
                          n5155 = Unbundle By Name(w4625) -> ("status"=w4624:bool)
                          n5156 = Search and Replace String(replace all?=TRUE ("replace all? (F)"), input string=w4614, search string="\\", replace string=w4611) -> (result string=w4610:string)  [unwired: 4 in, 3 out]
                          n5157 = case shown="True" w4624 {
                            tunnel: w4623 -> [w4627 w4629]
                            tunnel: [w4627 w4628] -> w4615
                            frame False {
                            }
                            frame True {
                              n5158 = Create Folder(path (use dialog)=w4629) -> (created path=w4628:path)  [unwired: 1 in, 3 out]
